vi "UpdateLineState.vi"(7 "DevControl 输入":refnum<class "DevControl.lvclass"> caption="DevClass", 8 "error in (no error)":errorcluster caption="错误输入（无错误）", 10 "¾€ów”µ“þ":refnum<vi>, 11 "¾€ów î‘B":refnum<vi>) -> (0 "error out":errorcluster caption="错误输出")   [LabVIEW 2012]
uses:
  Fun/Dev/SupportVi/DevState.ctl
  Fun/Dev/DevControl.lvclass
  Fun/Dev/SupportVi/LampState.ctl
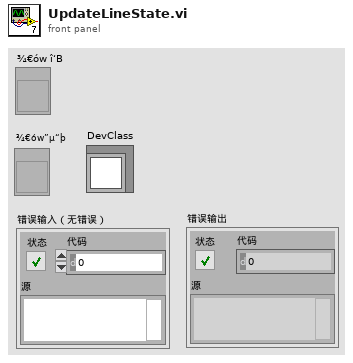
[diagram p1: front panel]
types:
  T1 = typedef "DevControl.lvclass/DevState.ctl" = enum16{"Shutdown", "PASS", "FAIL", "Idle", "Noresponse"}
  T2 = cluster{"Addr":u8, "name":string, "State":T1, "Retry":i32}[]
  T3 = typedef "DevControl.lvclass/LampState.ctl" = enum16{"üS+·äøQÆ÷", "¼t+·äøQÆ÷", "·äøQÆ÷", "È«œç", "全亮", "üS", "¾G", "¼t"}
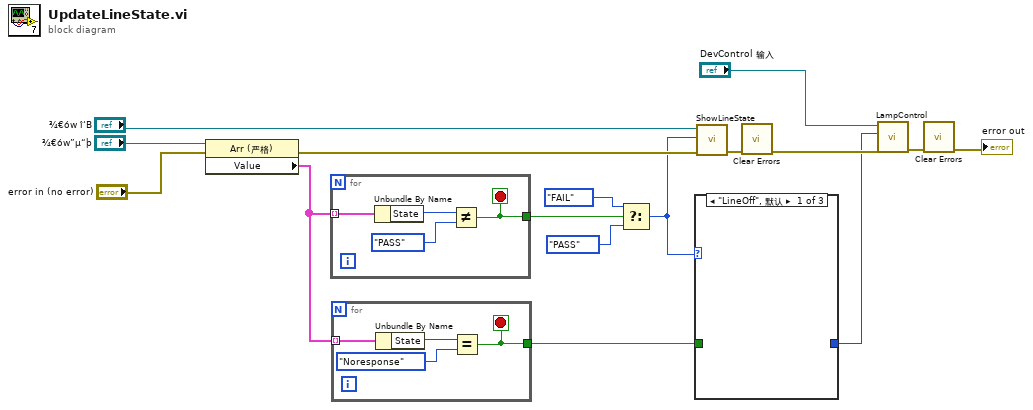
[diagram p0: block diagram]
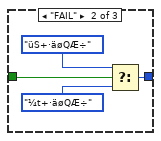
[diagram p2: hidden frame]
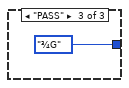
[diagram p3: hidden frame]
diagram:
  n1 = property class="Arr (严格)"(reference="¾€ów”µ“þ", error in="error in (no error)") -> (error out=w13:errorcluster, "Value"=w6:T2)  [unwired: 1 out]
  n2 = for {
    tunnel: w6 -> [w20] mode=indexing
    tunnel: [w17] -> w14
    stop <- w17 stop-if-true
    n3 = Unbundle By Name(w20) -> ("State"=w19:T1)
    n4 = Not Equal?(x=w19, y=DevState."PASS" ("State")) -> (x != y?=w17:bool)
  }
  n5 = for {
    tunnel: w6 -> [w24] mode=indexing
    tunnel: [w21] -> w2
    stop <- w21 stop-if-true
    n6 = Unbundle By Name(w24) -> ("State"=w23:T1)
    n7 = Equal?(x=w23, y=DevState."Noresponse" ("State")) -> (x = y?=w21:bool)
  }
  n8 = Select(t=enum16{"LineOff", "FAIL", "PASS"}."FAIL" ("LineState"), s=w14, f=enum16{"LineOff", "FAIL", "PASS"}."PASS" ("LineState")) -> (s? t:f=w5:enum16{"LineOff", "FAIL", "PASS"})
  n9 = case shown="\"LineOff\", 默认" w5 {
    tunnel: [_ w25 LampState."¾G" ("ÈýÉ«Ÿô î‘B")] -> w3
    tunnel: w2 -> [_ w28 _]
    frame "LineOff", Default {
    }
    frame "FAIL" {
      n10 = Select(t=LampState."üS+·äøQÆ÷" ("ÈýÉ«Ÿô î‘B"), s=w28, f=LampState."¼t+·äøQÆ÷" ("ÈýÉ«Ÿô î‘B")) -> (s? t:f=w25:T3)
    }
    frame "PASS" {
    }
  }
  n11 = call "ShowLineState.vi"("错误输入（无错误）"=w13, "LineState"=w5, "¾€ów î‘BÒýÓÃ"="¾€ów î‘B") -> ("错误输出"=w9:errorcluster)  [unwired: 8 in]
  n12 = call <vilib>:"Clear Errors.vi"("error in (no error)"=w9) -> ("error out"=w8:errorcluster)  [unwired: 6 in]
  n13 = call-dynamic "LampControl.vi"("error in (no error)"=w8, "ÈýÉ«Ÿô î‘B"=w3, "DevControl 输入"="DevControl 输入") -> ("error out"=w4:errorcluster)  [unwired: 7 in, 1 out]
  n14 = call <vilib>:"Clear Errors.vi"("error in (no error)"=w4) -> ("error out"=→"error out":errorcluster)  [unwired: 6 in]
